vi "Flush Data to Log File.vi"(8 "error in (no error)":errorcluster, 10 "Data Queue":T2, 11 "Logging Configuration":T1) -> (0 "error out":errorcluster)   [LabVIEW 2015, in "Logging.lvlib"]
doc: "Flush the data queue of any pending data and write it to the log file. Close the TDMS file reference."
uses:
  Logging.lvlib
  controls/Data queue.ctl
  Acquisition/Generic data packet.ctl
  My Graphs/Gps Map Graph coordinates.ctl
  Logging Configuration.ctl
  Acquisition/Acquisition.lvlib
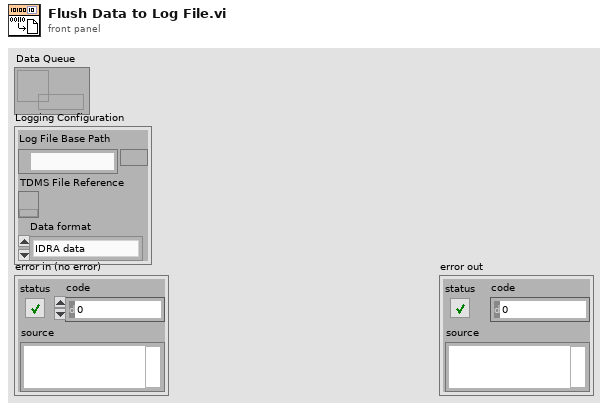
[diagram p1: front panel]
types:
  T1 = typedef "Logging.lvlib/Logging Configuration.ctl" = cluster{"Log File Base Path":path, "TDMS File Reference":refnum<k34>, "Data format":enum16{"IDRA data", "XAM data"}}
  T2 = typedef "Data queue.ctl" = refnum<queue>
  T3 = typedef "Acquisition.lvlib/Generic data packet.ctl" = cluster{"Content type":enum16{"None", "Telemetria", "GPS"}, "GPS":T4, "Telemetria":cluster{"Data format":enum16{"IDRA data", "XAM data"}, "Data":variant}}
  T4 = typedef "Gps Map Graph coordinates.ctl" = cluster{"Latitude":dbl, "Longitude":dbl}
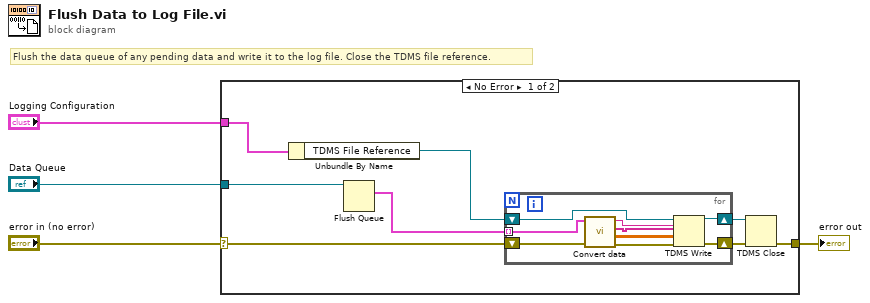
[diagram p0: block diagram]
diagram:
  # "Flush the data queue of any pending data and write it to the log file. Close the TDMS file reference."
  n1 = case shown="No Error" "error in (no error)" {
    selector: "error in (no error)" -> [w5 w22]
    tunnel: "Data Queue" -> [w8 _]
    tunnel: "Logging Configuration" -> [w7 _]
    tunnel: [w6 w22] -> w2
    frame No Error {
      n2 = Unbundle By Name(w7) -> ("TDMS File Reference"=w9:refnum<k34>)
      n3 = Flush Queue(queue=w8) -> (remaining elements=w12:T3[])  [unwired: 1 in, 2 out]
      n4 = for {
        shift-right: [w19] -> w10
        shift-left: w9 -> [w20]
        shift-right: [w21] -> w11
        shift-left: w5 -> [w17]
        tunnel: w12 -> [w18] mode=indexing
        n5 = call "Convert data.vi"("Error in"=w17, "Element in"=w18) -> ("Error out"=w16:errorcluster, "Data out"=w13:dbl[][], "Channels name"=w14:string[], "Content type"=w15:string)  [unwired: 6 in]
        n6 = TDMS Write(0:w20, 5:w15, 7:w14, 9:w13, 11:w16) -> (4:w19:refnum<k34>, 15:w21:errorcluster)  [unwired: 1 in, 2 out]
      }
      n7 = TDMS Close(8:w11, 11:w10) -> (0:w6:errorcluster)  [unwired: 1 out]
    }
    frame Error {
    }
  }
  "error out" <- w2
